vi "String_Voltage.vi"(11 "String":string="Set Voltage 5V at 5V/min, Sweep&meas") -> (2 "Rate":dbl, 3 "Voltage":dbl, 4 "V.Wait Stability":bool)   [LabVIEW 2017]
panel:
  out "subString":string
  # "Set Voltage 4.2V at 20V/min, Wait"
  # "Set Voltage 4.2V at 20V/min, NOWait"
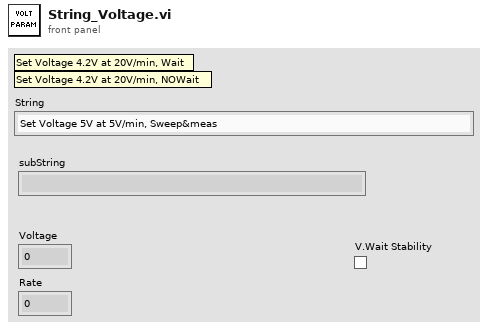
[diagram p1: front panel]
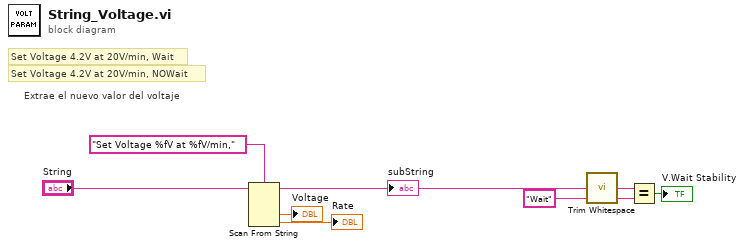
[diagram p0: block diagram]
diagram:
  # "Set Voltage 4.2V at 20V/min, NOWait"
  # "Set Voltage 4.2V at 20V/min, Wait"
  # "Extrae el nuevo valor del voltaje"
  n1 = Scan From String(format string="Set Voltage %fV at %fV/min,", input string="String") -> (remaining string=w1:string, output 1=→"Voltage":dbl, output 2=→"Rate":dbl)  [unwired: 4 in, 2 out]
  "subString" <- w1
  n2 = call <vilib>:"Trim Whitespace.vi"("string"=w1) -> ("trimmed string"=w2:string)  [unwired: 1 in]
  n3 = Equal?(x=w2, y="Wait" ("after substring")) -> (x = y?=→"V.Wait Stability":bool)
